vi "PH_PowerUnit_BaseClass.set GUI Refs.vi"(0 "i ref  in":refnum<vi>, 2 "Class":string, 3 "GUI Refs":T3, 5 "error in":errorcluster) -> (14 "i ref out":refnum<vi>, 19 "error out":errorcluster)   [LabVIEW 2014, in "PH_PowerUnit_BaseClass.lvlib"]
uses:
  PH_PowerUnit_BaseClass.lvlib
  PH_PowerUnit_BaseClass.GUI Refs to pack.ctl
  PH_PowerUnit_BaseClass.GUI Refs.ctl
  PH_PowerUnit_BaseClass.SM States.ctl
  PH_PSDBWriter/PH_PSDBWriter.lvlib
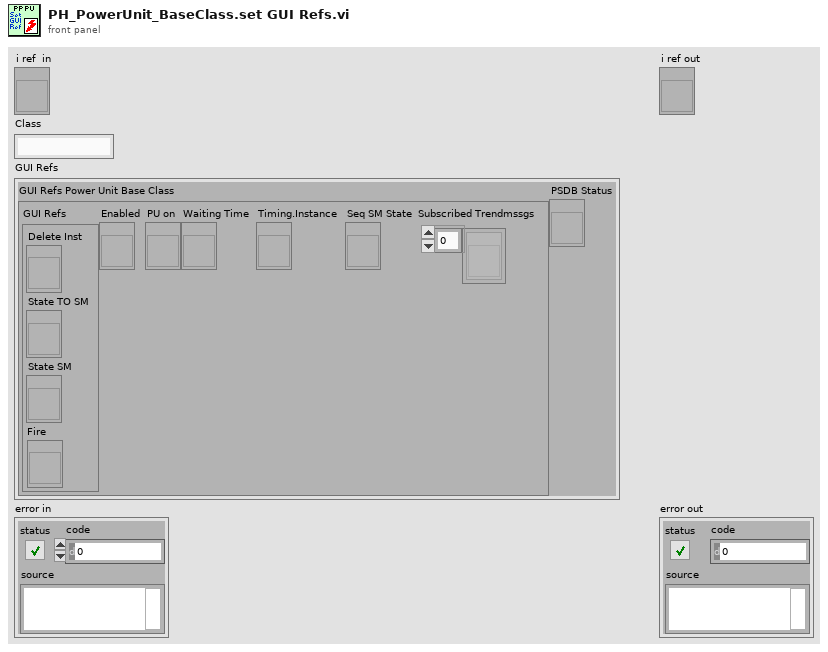
[diagram p1: front panel]
types:
  T1 = typedef "PH_PowerUnit_BaseClass.lvlib/PH_PowerUnit_BaseClass.GUI Refs to pack.ctl" = cluster{"GUI Refs":T2, "Enabled":refnum<vi>, "PU on":refnum<vi>, "Waiting Time":refnum<vi>, "Timing.Instance":refnum<vi>, "Seq SM State":refnum<vi>, "Subscribed Trendmssgs":refnum<vi>[]}
  T2 = typedef "PH_PowerUnit_BaseClass.lvlib/PH_PowerUnit_BaseClass.GUI Refs.ctl" = cluster{"Delete Inst":refnum<vi>, "State TO SM":refnum<vi>, "State SM":refnum<vi>, "Fire":refnum<vi>}
  T3 = cluster{"GUI Refs Power Unit Base Class":T1, "PSDB Status":refnum<vi>}
  T4 = typedef "PH_PowerUnit_BaseClass.lvlib/PH_PowerUnit_BaseClass.i attribute.ctl" = cluster{"Constructor finished":bool, "PU":cluster{"In use":bool, "Service ID in use":i32, "GUI Ref":refnum<vi>}, "Enabling":cluster{"State":T5, "GUI Ref":refnum<vi>}, "Timing":cluster{"Last Shot":dbl, "Time between Shots [Sec]":dbl, "Waiting Time over?":bool, "Service ID Waiting Time":i32, "GUI Ref":refnum<vi>, "Instance":cluster{"Status":T6, "linked?":bool, "GUI Ref":refnum<vi>}}, "Sequencer":cluster{"SM State":string, "GUI Ref":refnum<vi>, "linked":bool}, "Subscribed Trendmssgs":cluster{"Tagname":string, "Status":T6, "linked?":bool, "Shot Condition":T6, "GUI Ref":refnum<vi>}[], "PP PU":T7, "Default Voltage (V)":dbl, "GUI Refs":T2, "PSDB data":cluster{"Shot Voltage [V]":dbl, "State TO SM":T8, "Write 2 early":bool}, "State TO SM":T8}
  T5 = typedef "PH_SystemInformation.lvlib/PH_SystemInformationEnabling State.ctl" = i32
  T6 = typedef "PH_StatusHandler.lvlib/PH_StatusHandler.Status.ctl" = i16
  T7 = typedef "PH_PP_Common.lvlib/PH_PP_Common.PUs.ctl" = enum16{"no Info", "PA-19mm-1", "PA-19mm-2", "PA-45mm-PILC", "PA-45mm-MAIN", "MA-PU-1", "MA-PU-2", "MA-PU-3", "MA-PU-4", "MA-PU-5", "MA-PU-6", "MA-FR", "MA-PILC", "PA-45mm-DP"}
  T8 = typedef "PH_PowerUnit_BaseClass.lvlib/PH_PowerUnit_BaseClass.SM States.ctl" = enum16{".", "Stand by", "Switch PU on", "Configure", "Set Default Voltage", "Set STANDBY", "Set READY", "Wait for Shot Cmd", "Open Dump Rods", "Open Ross Relais", "Close Ross Relais", "Switch PSU on", "Switch PSU off", "Charge", "Switch GD Channel on", "Close Dump Rods", "Rods-TO", "RR-TO", "PSU-TO", "Trigger-TO"}
  T9 = cluster{"Tagname":string, "Status":T6, "linked?":bool, "Shot Condition":T6, "GUI Ref":refnum<vi>}[]
  T10 = cluster{"Tagname":string, "Status":T6, "linked?":bool, "Shot Condition":T6, "GUI Ref":refnum<vi>}
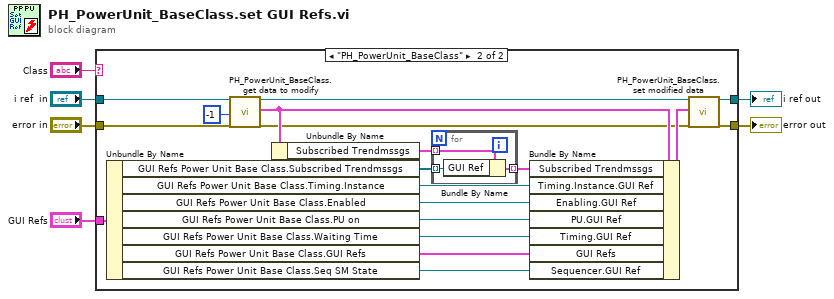
[diagram p0: block diagram]
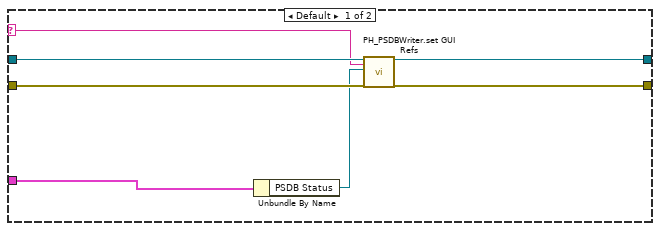
[diagram p2: hidden frame]
diagram:
  n1 = case shown="\"PH_PowerUnit_BaseClass\"" "Class" {
    selector: "Class" -> [w9 _]
    tunnel: [w11 w31] -> w2
    tunnel: [w12 w30] -> w3
    tunnel: "error in" -> [w10 w29]
    tunnel: "i ref  in" -> [w13 w28]
    tunnel: "GUI Refs" -> [w8 w21]
    frame Default {
      n2 = Unbundle By Name(w8) -> ("PSDB Status"=w7:refnum<vi>)
      n3 = call "PH_PSDBWriter.set GUI Refs.vi"("i ref in"=w13, "Class"=w9, "Ref PSDB Status"=w7, "error in"=w10) -> ("i ref out"=w12:refnum<vi>, "error out"=w11:errorcluster)  [unwired: 14 in]
    }
    frame "PH_PowerUnit_BaseClass" {
      n4 = Unbundle By Name(w21) -> ("GUI Refs Power Unit Base Class.Subscribed Trendmssgs"=w20:refnum<vi>[], "GUI Refs Power Unit Base Class.Timing.Instance"=w19:refnum<vi>, "GUI Refs Power Unit Base Class.Enabled"=w18:refnum<vi>, "GUI Refs Power Unit Base Class.PU on"=w17:refnum<vi>, "GUI Refs Power Unit Base Class.Waiting Time"=w16:refnum<vi>, "GUI Refs Power Unit Base Class.GUI Refs"=w15:T2, "GUI Refs Power Unit Base Class.Seq SM State"=w14:refnum<vi>)
      n5 = call "PH_PowerUnit_BaseClass.get data to modify.vi"("i ref in"=w28, "ms timeout (10000)"=-1, "error in (no error)"=w29) -> ("i ref out"=w26:refnum<vi>, "i attribute"=w32:T4, "error out"=w24:errorcluster)  [unwired: 13 in, 1 out]
      n6 = Unbundle By Name(w32) -> ("Subscribed Trendmssgs"=w22:T9)
      n7 = for {
        tunnel: w22 -> [w35] mode=indexing
        tunnel: [w34] -> w23 mode=indexing
        tunnel: w20 -> [w33] mode=indexing
        n8 = Bundle By Name(cluster=w35, "GUI Ref"=w33) -> (w34:T10)
      }
      n9 = Bundle By Name(cluster=w32, "Subscribed Trendmssgs"=w23, "Timing.Instance.GUI Ref"=w19, "Enabling.GUI Ref"=w18, "PU.GUI Ref"=w17, "Timing.GUI Ref"=w16, "GUI Refs"=w15, "Sequencer.GUI Ref"=w14) -> (w27:T4)
      n10 = call "PH_PowerUnit_BaseClass.set modified data.vi"("i ref in"=w26, "i attribute"=w27, "error in (no error)"=w24) -> ("i ref out"=w30:refnum<vi>, "error out"=w31:errorcluster)  [unwired: 15 in]
    }
  }
  "error out" <- w2
  "i ref out" <- w3
